vi "check.vi"(9 "帧头":u16=43605 format="%x", 11 "数据输入":u8[](array[numeric])) -> (2 "x与y?":bool, 3 "data输出":u8[](array[numeric]))   [LabVIEW 2012]
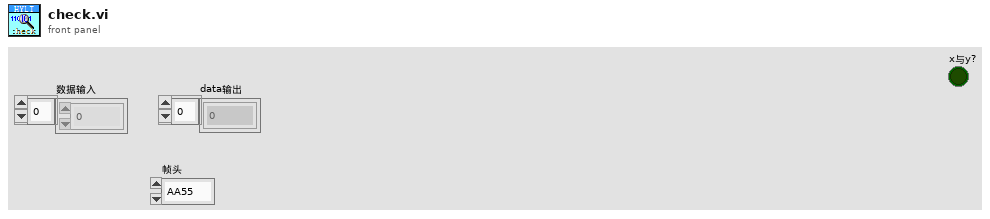
[diagram p1: front panel]
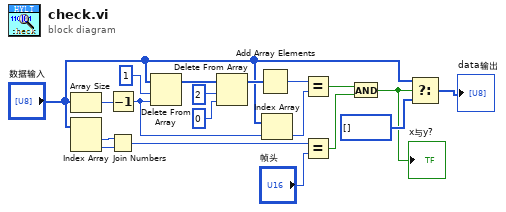
[diagram p0: block diagram]
diagram:
  n1 = Array Size(array="数据输入") -> (size(s)=w5:i32)
  n2 = Index Array(array="数据输入") -> (element #1=w10:u8, element #2=w9:u8)  [unwired: 2 in]
  n3 = Decrement(x=w5) -> (x-1=w4:i32)
  n4 = Join Numbers(hi=w10, lo=w9) -> ((hi.lo)=w11:u16)
  n5 = Delete From Array(array="数据输入", length=1 ("长度"), index=w4) -> (array with subset deleted=w18:u8[])  [unwired: 1 out]
  n6 = Delete From Array(array=w18, length=2 ("长度"), index=0 ("索引")) -> (array with subset deleted=w6:u8[])  [unwired: 1 out]
  n7 = Add Array Elements(numeric array=w6) -> (sum=w7:u8)
  n8 = Index Array(array="数据输入", index=w4) -> (element=w13:u8)
  n9 = Equal?(x=w7, y=w13) -> (x = y?=w14:bool)
  n10 = Equal?(x=w11, y="帧头") -> (x = y?=w15:bool)
  n11 = And(x=w14, y=w15) -> (x .and. y?=w8:bool)
  "x与y?" <- w8
  n12 = Select(t="数据输入", s=w8, f=u8[] []) -> (s? t:f=→"data输出":u8[])
